vi "PrincipalP11.vi"() -> ()   [LabVIEW 2018]
uses:
  EdosEntrada.ctl
  EdosPuente.ctl
  EdosSalida.ctl
panel:
  out "ListoSalir":bool
  out "H1Sal":bool
  out "H0Sal":bool
  out "BandSal":i32
  out "SalTime":dbl
  out "EdoSal":T1(ring)
  out "ClaseLeida":i32
  in  "Clase":i32(knob) scale=0.0..2.0
  out "H1Pte":bool
  out "H0Pte":bool
  out "BandPte":i32
  out "PteTime":dbl
  out "Puente":bool
  out "EdoPte":T2(ring)
  out "EntPiston":bool
  out "BandEnt":i32
  out "H1Ent":bool
  out "H0Ent":bool
  out "EntTime":dbl
  out "EdoEntrada":T3
  in  "P1":bool
  in  "P2":bool
  in  "P3":bool
  in  "S3":bool
  in  "S2":bool
  in  "S1":bool
  in  "E3":bool
  in  "E2":bool
  in  "E1":bool
  in  "stop":bool
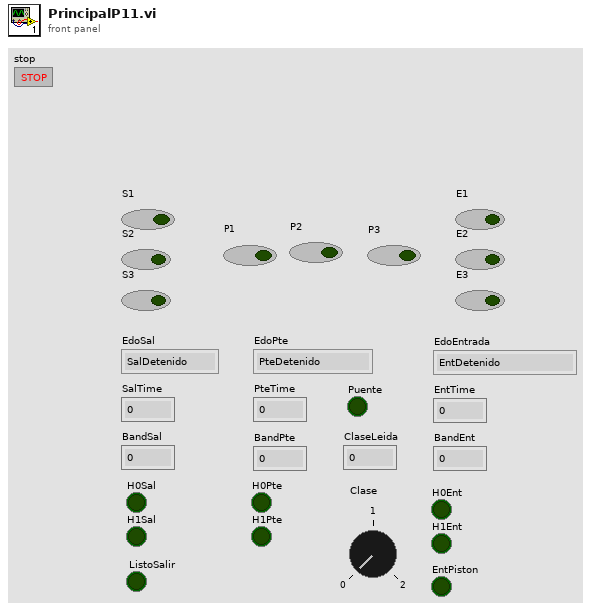
[diagram p1: front panel]
types:
  T1 = enum16{"SalDetenido", "SalPausa1", "SarDer", "SalIzq", "SalSal", "SalPausa2"}
  T2 = enum16{"PteDetenido", "PtePausa1", "PteMueveMitad", "PteAnaliza", "PteMueveSal", "PtePasa", "PtePausa2"}
  T3 = typedef "EdosEntrada.ctl" = enum16{"EntDetenido", "EntPausa1", "EntMueve", "EntPuente", "EntTransfiere", "EntPausa2"}
  T4 = typedef "EdosSalida.ctl" = enum16{"SalDetenido", "SalPausa1", "SarDer", "SalIzq", "SalSal", "SalPausa2"}
  T5 = typedef "EdosPuente.ctl" = enum16{"PteDetenido", "PtePausa1", "PteMueveMitad", "PteAnaliza", "PteMueveSal", "PtePasa", "PtePausa2"}
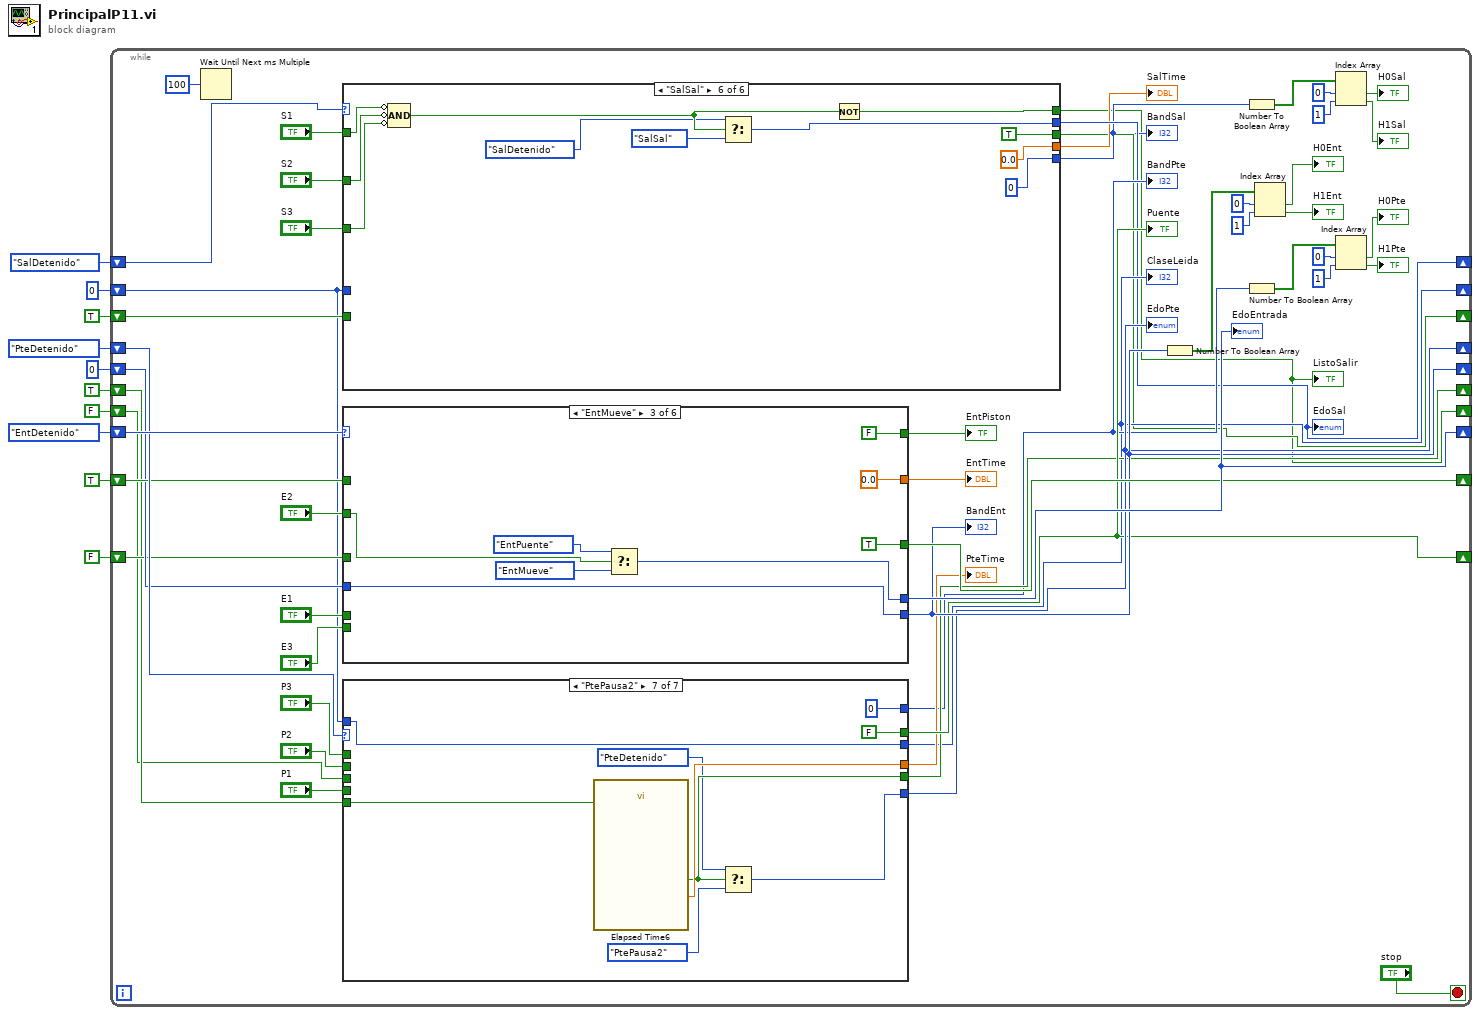
[diagram p0: block diagram]
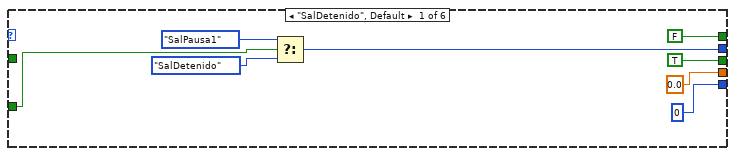
[diagram p2: hidden frame]
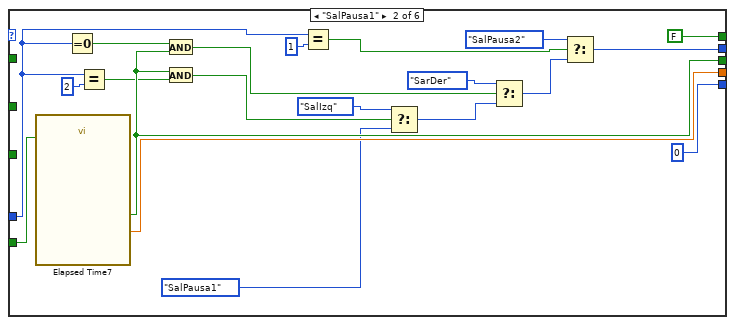
[diagram p3: hidden frame]
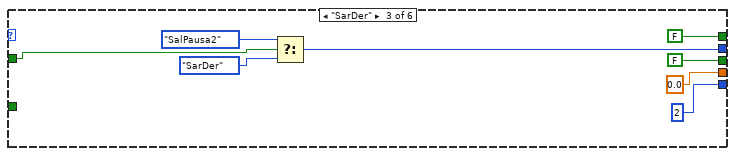
[diagram p4: hidden frame]
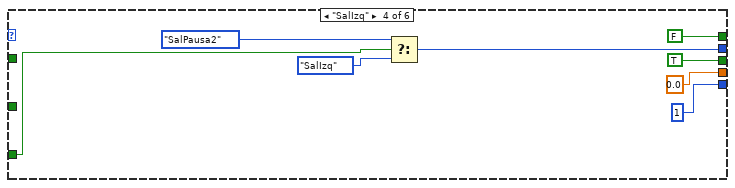
[diagram p5: hidden frame]
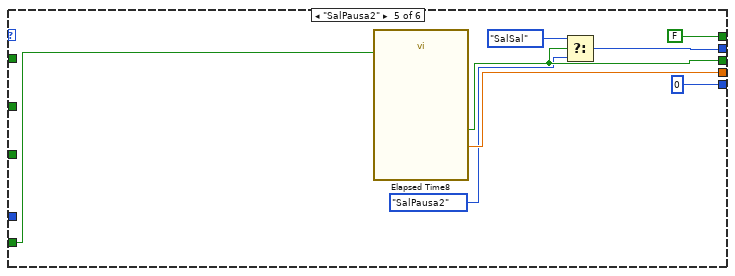
[diagram p6: hidden frame]
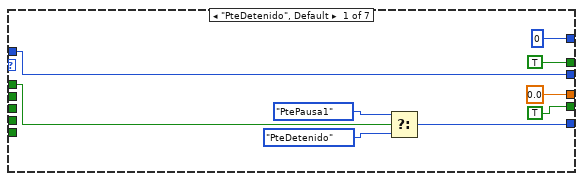
[diagram p7: hidden frame]
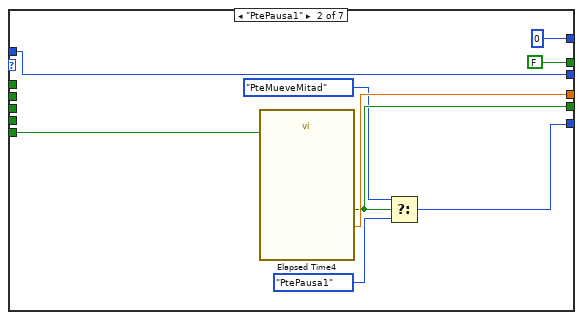
[diagram p8: hidden frame]
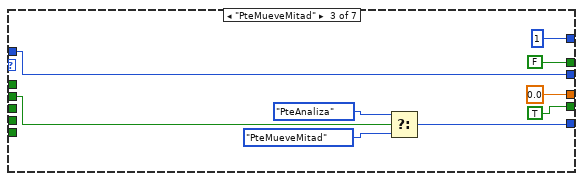
[diagram p9: hidden frame]
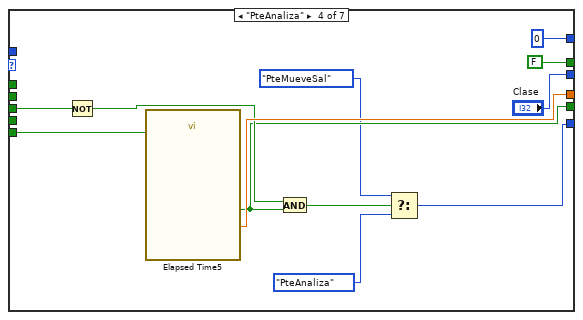
[diagram p10: hidden frame]
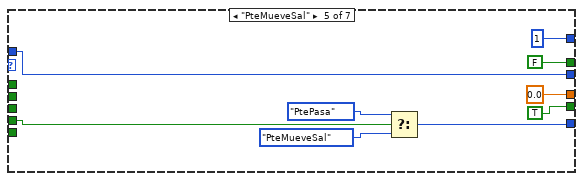
[diagram p11: hidden frame]
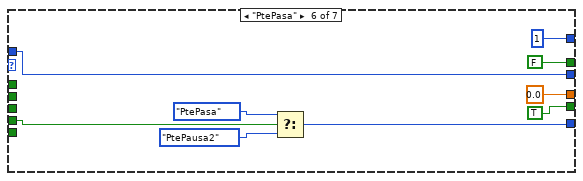
[diagram p12: hidden frame]
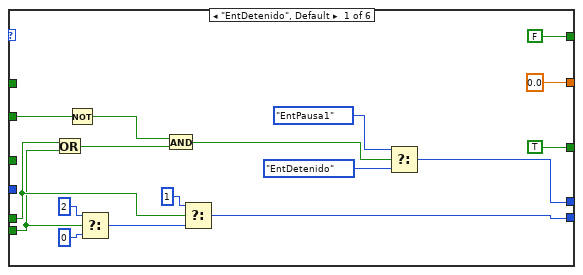
[diagram p13: hidden frame]
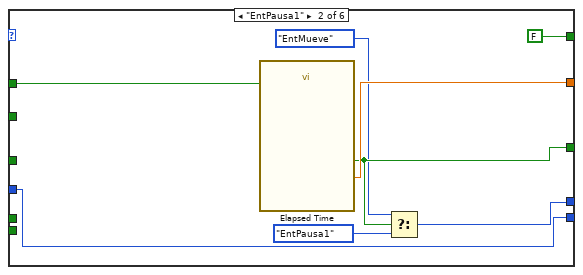
[diagram p14: hidden frame]
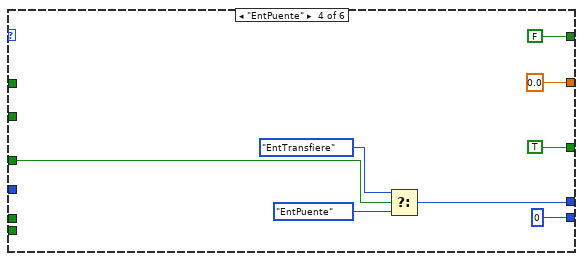
[diagram p15: hidden frame]
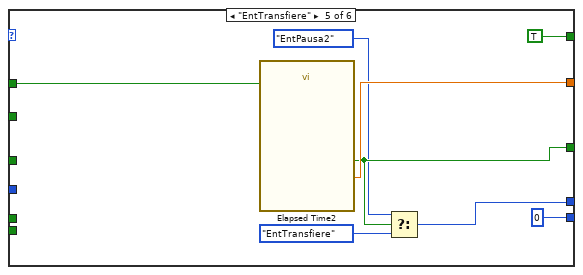
[diagram p16: hidden frame]
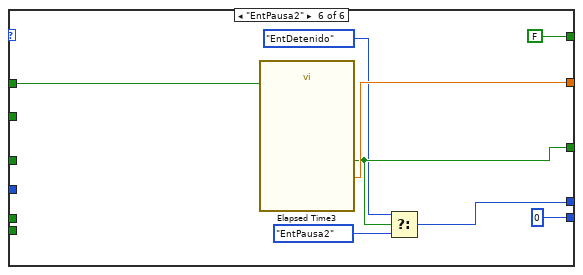
[diagram p17: hidden frame]
diagram:
  n1 = while {
    shift-right: [w54] -> _
    shift-left: EdosEntrada."EntDetenido" -> [w60]
    shift-right: [w41] -> _
    shift-left: EdosPuente."PteDetenido" -> [w59]
    shift-right: [w23] -> _
    shift-left: EdosSalida."SalDetenido" -> [w58]
    shift-right: [w51] -> _
    shift-left: TRUE -> [w52]
    shift-right: [w44] -> _
    shift-left: 0 -> [w50]
    shift-right: [w39] -> _
    shift-left: FALSE -> [w40]
    shift-right: [w37] -> _
    shift-left: TRUE -> [w38]
    shift-right: [w28] -> _
    shift-left: 0 -> [w19]
    shift-right: [w21] -> _
    shift-left: TRUE -> [w20]
    shift-right: [w11] -> _
    shift-left: FALSE -> [w12]
    stop <- "stop" stop-if-true
    n2 = Wait Until Next ms Multiple(millisecond multiple=u32 100) -> ()  [unwired: 1 out]
    n3 = case shown="\"SalSal\"" w58 {
      tunnel: "S1" -> [_ _ w96 _ _ w125]
      tunnel: "S2" -> [w70 _ _ _ _ w124]
      tunnel: "S3" -> [_ _ _ w106 _ w123]
      tunnel: [w69 w89 w95 w105 w110 w122] -> w23
      tunnel: [0.0 ("Elapsed Time (s)") w90 0.0 ("Elapsed Time (s)") 0.0 ("Elapsed Time (s)") w113 0.0 ("Elapsed Time (s)")] -> w22
      tunnel: [TRUE ("Time has Elapsed") w76 FALSE ("Time has Elapsed") TRUE ("Time has Elapsed") w111 TRUE ("Time has Elapsed")] -> w21
      tunnel: w20 -> [_ w88 _ _ w112 _]
      tunnel: w19 -> [_ w82 _ _ _ _]
      tunnel: [0 0 2 1 0 0] -> w18
      tunnel: [FALSE FALSE FALSE FALSE FALSE w117] -> w11
      frame "SalDetenido", Default {
        n4 = Select(t=EdosSalida."SalPausa1", s=w70, f=EdosSalida."SalDetenido") -> (s? t:f=w69:T4)
      }
      frame "SalPausa1" {
        n5 = call "Elapsed Time7"("Reset"=w88) -> ("Elapsed Time (s)"=w90:dbl, "Time has Elapsed"=w76:bool)  [unwired: 11 in, 6 out]
        n6 = Equal To 0?(x=w82) -> (x = 0?=w85:bool)
        n7 = Equal?(x=w82, y=2) -> (x = y?=w75:bool)
        n8 = And(x=w85, y=w76) -> (x .and. y?=w79:bool)
        n9 = And(x=w76, y=w75) -> (x .and. y?=w78:bool)
        n10 = Equal?(x=w82, y=1) -> (x = y?=w80:bool)
        n11 = Select(t=EdosSalida."SalIzq", s=w78, f=EdosSalida."SalPausa1") -> (s? t:f=w83:T4)
        n12 = Select(t=EdosSalida."SarDer", s=w79, f=w83) -> (s? t:f=w87:T4)
        n13 = Select(t=EdosSalida."SalPausa2", s=w80, f=w87) -> (s? t:f=w89:T4)
      }
      frame "SarDer" {
        n14 = Select(t=EdosSalida."SalPausa2", s=w96, f=EdosSalida."SarDer") -> (s? t:f=w95:T4)
      }
      frame "SalIzq" {
        n15 = Select(t=EdosSalida."SalPausa2", s=w106, f=EdosSalida."SalIzq") -> (s? t:f=w105:T4)
      }
      frame "SalPausa2" {
        n16 = call "Elapsed Time8"("Reset"=w112) -> ("Elapsed Time (s)"=w113:dbl, "Time has Elapsed"=w111:bool)  [unwired: 11 in, 6 out]
        n17 = Select(t=EdosSalida."SalSal", s=w111, f=EdosSalida."SalPausa2") -> (s? t:f=w110:T4)
      }
      frame "SalSal" {
        n18 = Compound Arithmetic op=AND(invert w125, invert w124, invert w123) -> (w118:bool)
        n19 = Select(t=EdosSalida."SalDetenido", s=w118, f=EdosSalida."SalSal") -> (s? t:f=w122:T4)
        n20 = Not(x=w118) -> (.not. x?=w117:bool)
      }
    }
    "EdoSal" <- w23
    "SalTime" <- w22
    "BandSal" <- w18
    "ListoSalir" <- w11
    n21 = case shown="\"EntMueve\"" w60 {
      tunnel: "E2" -> [w208 _ w224 _ _ _]
      tunnel: "E1" -> [w199 _ _ _ _ _]
      tunnel: "E3" -> [w196 _ _ _ _ _]
      tunnel: [w202 w211 w221 w228 w234 w241] -> w54
      tunnel: [0.0 ("Elapsed Time (s)") w216 0.0 ("Elapsed Time (s)") 0.0 ("Elapsed Time (s)") w240 w248] -> w53
      tunnel: w52 -> [_ w215 _ _ w239 w247]
      tunnel: [TRUE ("Time has Elapsed") w214 TRUE ("Time has Elapsed") TRUE ("Time has Elapsed") w237 w245] -> w51
      tunnel: w50 -> [_ w210 w218 _ _ _]
      tunnel: [w193 w210 w218 0 ("f") 0 ("f") 0 ("f")] -> w44
      tunnel: w40 -> [_ _ _ w231 _ _]
      tunnel: [FALSE FALSE FALSE FALSE TRUE FALSE] -> w43
      frame "EntDetenido", Default {
        n22 = Or(x=w199, y=w196) -> (x .or. y?=w206:bool)
        n23 = Not(x=w208) -> (.not. x?=w207:bool)
        n24 = Select(t=2, s=w196, f=0) -> (s? t:f=w197:i32)
        n25 = And(x=w207, y=w206) -> (x .and. y?=w205:bool)
        n26 = Select(t=1, s=w199, f=w197) -> (s? t:f=w193:i32)
        n27 = Select(t=EdosEntrada."EntPausa1", s=w205, f=EdosEntrada."EntDetenido") -> (s? t:f=w202:T3)
      }
      frame "EntPausa1" {
        n28 = call "Elapsed Time"("Reset"=w215) -> ("Elapsed Time (s)"=w216:dbl, "Time has Elapsed"=w214:bool)  [unwired: 11 in, 6 out]
        n29 = Select(t=EdosEntrada."EntMueve", s=w214, f=EdosEntrada."EntPausa1") -> (s? t:f=w211:T3)
      }
      frame "EntMueve" {
        n30 = Select(t=EdosEntrada."EntPuente", s=w224, f=EdosEntrada."EntMueve") -> (s? t:f=w221:T3)
      }
      frame "EntPuente" {
        n31 = Select(t=EdosEntrada."EntTransfiere", s=w231, f=EdosEntrada."EntPuente") -> (s? t:f=w228:T3)
      }
      frame "EntTransfiere" {
        n32 = call "Elapsed Time2"("Reset"=w239) -> ("Elapsed Time (s)"=w240:dbl, "Time has Elapsed"=w237:bool)  [unwired: 11 in, 6 out]
        n33 = Select(t=EdosEntrada."EntPausa2", s=w237, f=EdosEntrada."EntTransfiere") -> (s? t:f=w234:T3)
      }
      frame "EntPausa2" {
        n34 = call "Elapsed Time3"("Reset"=w247) -> ("Elapsed Time (s)"=w248:dbl, "Time has Elapsed"=w245:bool)  [unwired: 11 in, 6 out]
        n35 = Select(t=EdosEntrada."EntDetenido", s=w245, f=EdosEntrada."EntPausa2") -> (s? t:f=w241:T3)
      }
    }
    "EdoEntrada" <- w54
    "EntTime" <- w53
    "BandEnt" <- w44
    "EntPiston" <- w43
    n36 = case shown="\"PtePausa2\"" w59 {
      tunnel: "P3" -> [w134 _ _ _ _ _ _]
      tunnel: [w133 w139 w148 w160 w168 w181 w186] -> w41
      tunnel: [TRUE FALSE FALSE FALSE FALSE FALSE FALSE] -> w39
      tunnel: w38 -> [_ w143 _ w161 _ _ w189]
      tunnel: [TRUE ("Time has Elapsed") w140 TRUE ("Time has Elapsed") w156 TRUE ("Time has Elapsed") TRUE ("Time has Elapsed") w187] -> w37
      tunnel: [0.0 ("Elapsed Time (s)") w141 0.0 ("Elapsed Time (s)") w163 0.0 ("Elapsed Time (s)") 0.0 ("Elapsed Time (s)") w191] -> w36
      tunnel: "P2" -> [_ _ w149 _ _ _ _]
      tunnel: [0 0 1 0 1 1 0] -> w34
      tunnel: w19 -> [w128 w137 w146 _ w173 w177 w185]
      tunnel: [w128 w137 w146 "Clase" w173 w177 w185] -> w28
      tunnel: "P1" -> [_ _ _ _ w169 w182 _]
      tunnel: w12 -> [_ _ _ w158 _ _ _]
      frame "PteDetenido", Default {
        n37 = Select(t=EdosPuente."PtePausa1", s=w134, f=EdosPuente."PteDetenido") -> (s? t:f=w133:T5)
      }
      frame "PtePausa1" {
        n38 = call "Elapsed Time4"("Reset"=w143) -> ("Elapsed Time (s)"=w141:dbl, "Time has Elapsed"=w140:bool)  [unwired: 11 in, 6 out]
        n39 = Select(t=EdosPuente."PteMueveMitad", s=w140, f=EdosPuente."PtePausa1") -> (s? t:f=w139:T5)
      }
      frame "PteMueveMitad" {
        n40 = Select(t=EdosPuente."PteAnaliza", s=w149, f=EdosPuente."PteMueveMitad") -> (s? t:f=w148:T5)
      }
      frame "PteAnaliza" {
        n41 = Not(x=w158) -> (.not. x?=w157:bool)
        n42 = call "Elapsed Time5"("Reset"=w161) -> ("Elapsed Time (s)"=w163:dbl, "Time has Elapsed"=w156:bool)  [unwired: 11 in, 6 out]
        n43 = And(x=w157, y=w156) -> (x .and. y?=w155:bool)
        n44 = Select(t=EdosPuente."PteMueveSal", s=w155, f=EdosPuente."PteAnaliza") -> (s? t:f=w160:T5)
      }
      frame "PteMueveSal" {
        n45 = Select(t=EdosPuente."PtePasa", s=w169, f=EdosPuente."PteMueveSal") -> (s? t:f=w168:T5)
      }
      frame "PtePasa" {
        n46 = Select(t=EdosPuente."PtePasa", s=w182, f=EdosPuente."PtePausa2") -> (s? t:f=w181:T5)
      }
      frame "PtePausa2" {
        n47 = call "Elapsed Time6"("Reset"=w189) -> ("Elapsed Time (s)"=w191:dbl, "Time has Elapsed"=w187:bool)  [unwired: 11 in, 6 out]
        n48 = Select(t=EdosPuente."PteDetenido", s=w187, f=EdosPuente."PtePausa2") -> (s? t:f=w186:T5)
      }
    }
    "EdoPte" <- w41
    "Puente" <- w39
    "PteTime" <- w36
    "BandPte" <- w34
    "ClaseLeida" <- w28
    n49 = Number To Boolean Array(number=w44) -> (Boolean array=w49:bool[])
    n50 = Number To Boolean Array(number=w18) -> (Boolean array=w17:bool[])
    n51 = Number To Boolean Array(number=w34) -> (Boolean array=w33:bool[])
    n52 = Index Array(array=w49, index #1=0 ("index"), index #2=1 ("index")) -> (element #1=→"H0Ent":bool, element #2=→"H1Ent":bool)
    n53 = Index Array(array=w17, index #1=0 ("index"), index #2=1 ("index")) -> (element #1=→"H0Sal":bool, element #2=→"H1Sal":bool)
    n54 = Index Array(array=w33, index #1=0 ("index"), index #2=1 ("index")) -> (element #1=→"H0Pte":bool, element #2=→"H1Pte":bool)
  }
